vi "RANDOM_RANGE.vi"(10 "value_low":dbl format="%.2f", 11 "value_high":dbl=1.0 format="%.2f") -> (3 "Value":dbl format="%.2f")   [LabVIEW 2016]
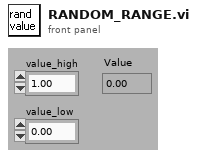
[diagram p1: front panel]
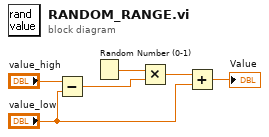
[diagram p0: block diagram]
diagram:
  n1 = Subtract(x="value_high", y="value_low") -> (x-y=w4:dbl)
  n2 = Random Number (0-1)() -> (number: 0 to 1=w5:dbl)
  n3 = Multiply(x=w5, y=w4) -> (x*y=w3:dbl)
  n4 = Add(x=w3, y="value_low") -> (x+y=→"Value":dbl)
